vi "updatePIDs.vi"(11 "MainTalon":T1={"DeviceStatus"={"status"=FALSE, "code"=0, "source"=""}, "Type"=enum."PWM", "PWM"={"PWM Channel"=enum."PWM 1", "DeadBand"={"Name"="", "maxPositivePwm"=0, "minPositivePwm"=0, "centerPwm"=0, "maxNegativePwm"=0, "minNegativePwm"=0, "angularRange"=0}}, "CAN"={"Device Number"=0, "SetOutput VI Ref"=variant(enum8{"Percent VBus", "Current", "Speed", "Position", "Voltage"} enum."Percent VBus"), "GetOutput VI Ref"=variant(refnum<k1> refnum), "Enable VI Ref"=variant(dbl 12.0), "Disable VI Ref"=variant(enum8{"Percent VBus", "Speed", "Position", "Slave", "Unchanged / Invalid", "Voltage Compensation", "Current", "Motion Profile"} enum."Percent VBus"), "Data"=variant}, "Invert"=FALSE, "DIO PWM"={"PWM \"Enable\" Channel"=enum."Invalid", "DIOChannel"=enum."Invalid", "PWM Rate"=0.0}}) -> ()   [LabVIEW 2018]
uses:
  <vilib>/Rock Robotics/WPI/MotorControl/WPI_MotorControlDeviceRef.ctl
  <vilib>/Rock Robotics/WPI/MotorControl/WPI_MotorControlType.ctl
  <vilib>/Rock Robotics/SystemInterfaces/DIO/FPGA_DIOPWMChannel.ctl
  <vilib>/Rock Robotics/WPI/PWM/WPI_PWMDeadband.ctl
  <vilib>/Rock Robotics/SystemInterfaces/DIO/FPGA_DIOChannel.ctl
  Constants.vi
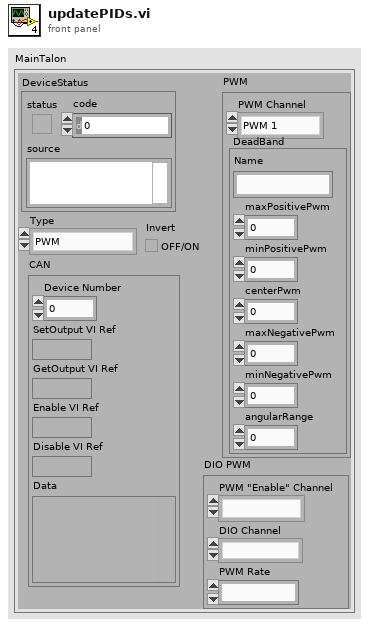
[diagram p1: front panel]
types:
  T1 = typedef "WPI_MotorControlDeviceRef.ctl" = cluster{"DeviceStatus":errorcluster, "Type":T2, "PWM":cluster{"PWM Channel":T3, "DeadBand":T4}, "CAN":cluster{"Device Number":u8, "SetOutput VI Ref":variant, "GetOutput VI Ref":variant, "Enable VI Ref":variant, "Disable VI Ref":variant, "Data":variant}, "Invert":bool, "DIO PWM":cluster{"PWM \"Enable\" Channel":T3, "DIOChannel":T5, "PWM Rate":dbl}}
  T2 = typedef "WPI_MotorControlType.ctl" = enum16{"PWM", "CAN", "DIO PWM"}
  T3 = typedef "FPGA_DIOPWMChannel.ctl" = enum8{"PWM 0", "PWM 1", "PWM 2", "PWM 3", "PWM 4", "PWM 5", "PWM 6", "PWM 7", "PWM 8", "PWM 9", "PWM MXP 0", "PWM MXP 1", "PWM MXP 2", "PWM MXP 3", "PWM MXP 4", "PWM MXP 5", "PWM MXP 6", "PWM MXP 7", "PWM MXP 8", "PWM MXP 9", "Invalid"}
  T4 = typedef "WPI_PWMDeadband.ctl" = cluster{"Name":string, "maxPositivePwm":i32, "minPositivePwm":i32, "centerPwm":i32, "maxNegativePwm":i32, "minNegativePwm":i32, "angularRange":u16}
  T5 = typedef "FPGA_DIOChannel.ctl" = enum8{"DIO 0", "DIO 1", "DIO 2", "DIO 3", "DIO 4", "DIO 5", "DIO 6", "DIO 7", "DIO 8", "DIO 9", "DIO MXP 0", "DIO MXP 1", "DIO MXP 2", "DIO MXP 3", "DIO MXP 4", "DIO MXP 5", "DIO MXP 6", "DIO MXP 7", "DIO MXP 8", "DIO MXP 9", "DIO MXP 10", "DIO MXP 11", "DIO MXP 12", "DIO MXP 13", "DIO MXP 14", "DIO MXP 15", "SPI Port CS1", "SPI Port CS2", "SPI Port CS3", "SPI Port MISO", "SPI Port MOSI", "Invalid"}
  T6 = cluster{"kP":dbl, "kI ":dbl, "kD":dbl, "kF":dbl, "I Zone":dbl, "Peak Out":dbl}
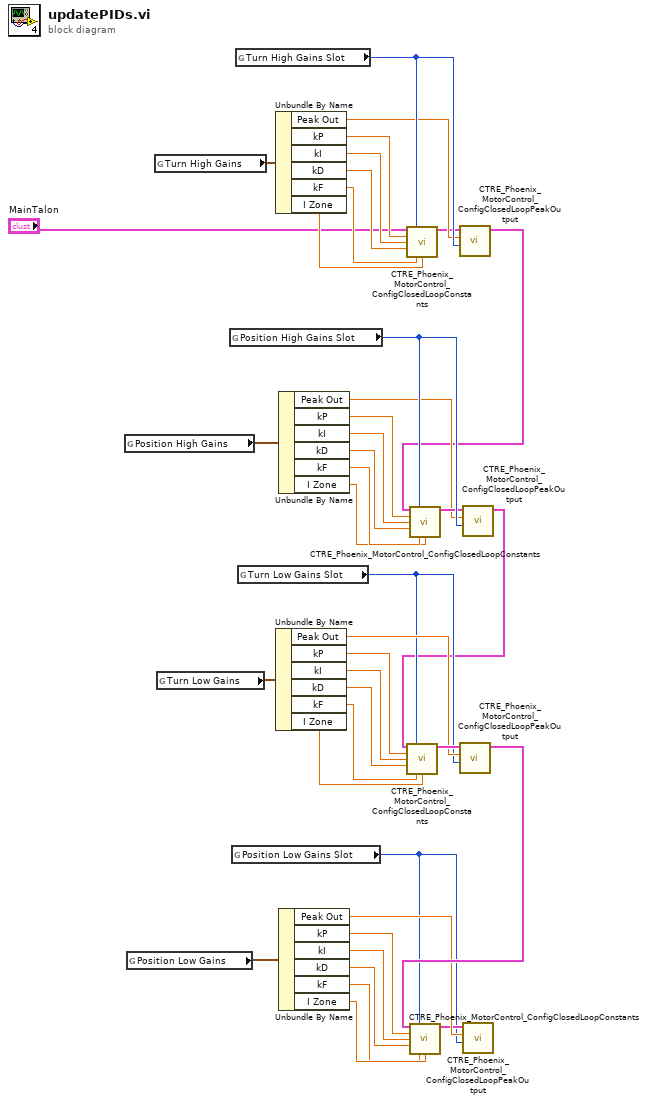
[diagram p0: block diagram]
diagram:
  n1 = global read "Constants.vi" "Position High Gains"() -> (w30:T6)
  n2 = global read "Constants.vi" "Position Low Gains"() -> (w12:T6)
  n3 = global read "Constants.vi" "Turn High Gains"() -> (w31:T6)
  n4 = global read "Constants.vi" "Turn Low Gains"() -> (w11:T6)
  n5 = global read "Constants.vi" "Position High Gains Slot"() -> (w39:i32)
  n6 = global read "Constants.vi" "Position Low Gains Slot"() -> (w3:i32)
  n7 = global read "Constants.vi" "Turn High Gains Slot"() -> (w40:i32)
  n8 = global read "Constants.vi" "Turn Low Gains Slot"() -> (w2:i32)
  n9 = Unbundle By Name(w31) -> ("Peak Out"=w38:dbl, "kP"=w32:dbl, "kI"=w33:dbl, "kD"=w34:dbl, "kF"=w35:dbl, "I Zone"=w36:dbl)
  n10 = Unbundle By Name(w11) -> ("Peak Out"=w4:dbl, "kP"=w10:dbl, "kI"=w9:dbl, "kD"=w8:dbl, "kF"=w7:dbl, "I Zone"=w6:dbl)
  n11 = Unbundle By Name(w30) -> ("Peak Out"=w23:dbl, "kP"=w29:dbl, "kI"=w28:dbl, "kD"=w27:dbl, "kF"=w26:dbl, "I Zone"=w25:dbl)
  n12 = Unbundle By Name(w12) -> ("Peak Out"=w19:dbl, "kP"=w13:dbl, "kI"=w14:dbl, "kD"=w15:dbl, "kF"=w16:dbl, "I Zone"=w17:dbl)
  n13 = call <vilib>:"CTRE_Phoenix_MotorControl_ConfigClosedLoopConstants.vi"("PhoenixMotorControlDevRef"="MainTalon", "slotIdx"=w40, "P"=w32, "I"=w33, "D"=w34, "F"=w35, "I Zone"=w36) -> ("PhoenixMotorControlDevRef"=w37:T1)  [unwired: 7 in, 1 out]
  n14 = call <vilib>:"CTRE_Phoenix_MotorControl_ConfigClosedLoopPeakOutput.vi"("slotIdx"=w40, "peakOutput"=w38, "PhoenixMotorControlDevRef"=w37) -> ("PhoenixMotorControlDevRef"=w22:T1)  [unwired: 7 in, 1 out]
  n15 = call <vilib>:"CTRE_Phoenix_MotorControl_ConfigClosedLoopConstants.vi"("PhoenixMotorControlDevRef"=w22, "slotIdx"=w39, "P"=w29, "I"=w28, "D"=w27, "F"=w26, "I Zone"=w25) -> ("PhoenixMotorControlDevRef"=w24:T1)  [unwired: 7 in, 1 out]
  n16 = call <vilib>:"CTRE_Phoenix_MotorControl_ConfigClosedLoopPeakOutput.vi"("slotIdx"=w39, "peakOutput"=w23, "PhoenixMotorControlDevRef"=w24) -> ("PhoenixMotorControlDevRef"=w1:T1)  [unwired: 7 in, 1 out]
  n17 = call <vilib>:"CTRE_Phoenix_MotorControl_ConfigClosedLoopConstants.vi"("PhoenixMotorControlDevRef"=w1, "slotIdx"=w2, "P"=w10, "I"=w9, "D"=w8, "F"=w7, "I Zone"=w6) -> ("PhoenixMotorControlDevRef"=w5:T1)  [unwired: 7 in, 1 out]
  n18 = call <vilib>:"CTRE_Phoenix_MotorControl_ConfigClosedLoopPeakOutput.vi"("slotIdx"=w2, "peakOutput"=w4, "PhoenixMotorControlDevRef"=w5) -> ("PhoenixMotorControlDevRef"=w20:T1)  [unwired: 7 in, 1 out]
  n19 = call <vilib>:"CTRE_Phoenix_MotorControl_ConfigClosedLoopConstants.vi"("PhoenixMotorControlDevRef"=w20, "slotIdx"=w3, "P"=w13, "I"=w14, "D"=w15, "F"=w16, "I Zone"=w17) -> ("PhoenixMotorControlDevRef"=w18:T1)  [unwired: 7 in, 1 out]
  n20 = call <vilib>:"CTRE_Phoenix_MotorControl_ConfigClosedLoopPeakOutput.vi"("slotIdx"=w3, "peakOutput"=w19, "PhoenixMotorControlDevRef"=w18) -> ()  [unwired: 7 in, 2 out]
